vi "Read Name core.vi"(11 "Build Item in":refnum<class "Run Tests Step.lvclass">) -> (2 "Name":string)   [LabVIEW 2019, in "Caraya Library.lvlib" / "Run Tests Step.lvclass"]
doc: "Gets the name for the build step\n\nCopyright: MGI 2016\nAuthor: Derek Trepanier"
uses:
  Run Tests Step.lvclass
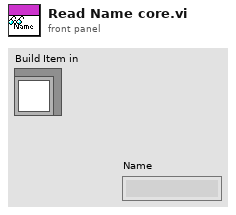
[diagram p1: front panel]
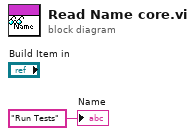
[diagram p0: block diagram]
diagram:
  "Name" <- "Run Tests" ("Name")
